vi "get voltage range ring.vi"(8 "error in (no error)":errorcluster caption="에러 입력(에러 없음)", 11 "DW7914 입력":refnum<class "DW7914.lvclass">) -> (0 "error out":errorcluster caption="에러 출력", 1 "caption":string="VD Clamp", 2 "strings & values":T1=[{"String"="0.00V", "Value"=0.0}, {"String"="0.04V", "Value"=0.04}, {"String"="0.08V", "Value"=0.08}, {"String"="0.12V", "Value"=0.12}, {"String"="0.16V", "Value"=0.16}, {"String"="0.20V", "Value"=0.2}, {"String"="0.24V", "Value"=0.24}, {"String"="0.28V", "Value"=0.28}, {"String"="0.32V", "Value"=0.32}, {"String"="0.36V", "Value"=0.36}, {"String"="0.40V", "Value"=0.4}, {"String"="0.44V", "Value"=0.44}, {"String"="0.48V", "Value"=0.48}, {"String"="0.52V", "Value"=0.52}, {"String"="0.56V", "Value"=0.56}, {"String"="0.60V", "Value"=0.6}, {"String"="0.64V", "Value"=0.64}, {"String"="0.68V", "Value"=0.68}, {"String"="0.72V", "Value"=0.72}, {"String"="0.76V", "Value"=0.76}, {"String"="0.80V", "Value"=0.8}, {"String"="0.84V", "Value"=0.84}, {"String"="0.88V", "Value"=0.88}, {"String"="0.92V", "Value"=0.92}, {"String"="0.96V", "Value"=0.96}, {"String"="1.00V", "Value"=1.0}, {"String"="1.04V", "Value"=1.04}, {"String"="1.08V", "Value"=1.08}, {"String"="1.12V", "Value"=1.12}, {"String"="1.16V", "Value"=1.16}, {"String"="1.20V", "Value"=1.2}, {"String"="1.24V", "Value"=1.24}, {"String"="1.28V", "Value"=1.28}, {"String"="1.32V", "Value"=1.32}, {"String"="1.36V", "Value"=1.36}, {"String"="1.40V", "Value"=1.4}, {"String"="1.44V", "Value"=1.44}, {"String"="1.48V", "Value"=1.48}, {"String"="1.52V", "Value"=1.52}, {"String"="1.56V", "Value"=1.56}, {"String"="1.60V", "Value"=1.6}, {"String"="1.64V", "Value"=1.64}, {"String"="1.68V", "Value"=1.68}, {"String"="1.72V", "Value"=1.72}, {"String"="1.76V", "Value"=1.76}, {"String"="1.80V", "Value"=1.8}, {"String"="1.84V", "Value"=1.84}, {"String"="1.88V", "Value"=1.88}, {"String"="1.92V", "Value"=1.92}, {"String"="1.96V", "Value"=1.96}, {"String"="2.00V", "Value"=2.0}, {"String"="2.04V", "Value"=2.04}, {"String"="2.08V", "Value"=2.08}, {"String"="2.12V", "Value"=2.12}, {"String"="2.16V", "Value"=2.16}, {"String"="2.20V", "Value"=2.2}, {"String"="2.24V", "Value"=2.24}, {"String"="2.28V", "Value"=2.28}, {"String"="2.32V", "Value"=2.32}, {"String"="2.36V", "Value"=2.36}, {"String"="2.40V", "Value"=2.4}, {"String"="2.44V", "Value"=2.44}, {"String"="2.48V", "Value"=2.48}, {"String"="2.52V", "Value"=2.52}, {"String"="2.56V", "Value"=2.56}, {"String"="2.60V", "Value"=2.6}, {"String"="2.64V", "Value"=2.64}, {"String"="2.68V", "Value"=2.68}, {"String"="2.72V", "Value"=2.72}, {"String"="2.76V", "Value"=2.76}, {"String"="2.80V", "Value"=2.8}, {"String"="2.84V", "Value"=2.84}, {"String"="2.88V", "Value"=2.88}, {"String"="2.92V", "Value"=2.92}, {"String"="2.96V", "Value"=2.96}, {"String"="3.00V", "Value"=3.0}, {"String"="3.04V", "Value"=3.04}, {"String"="3.08V", "Value"=3.08}, {"String"="3.12V", "Value"=3.12}, {"String"="3.16V", "Value"=3.16}, {"String"="3.20V", "Value"=3.2}, {"String"="3.24V", "Value"=3.24}, {"String"="3.28V", "Value"=3.28}, {"String"="3.32V", "Value"=3.32}, {"String"="3.36V", "Value"=3.36}, {"String"="3.40V", "Value"=3.4}, {"String"="3.44V", "Value"=3.44}, {"String"="3.48V", "Value"=3.48}, {"String"="3.52V", "Value"=3.52}, {"String"="3.56V", "Value"=3.56}, {"String"="3.60V", "Value"=3.6}, {"String"="3.64V", "Value"=3.64}, {"String"="3.68V", "Value"=3.68}, {"String"="3.72V", "Value"=3.72}, {"String"="3.76V", "Value"=3.76}, {"String"="3.80V", "Value"=3.8}, {"String"="3.84V", "Value"=3.84}, {"String"="3.88V", "Value"=3.88}, {"String"="3.92V", "Value"=3.92}, {"String"="3.96V", "Value"=3.96}, {"String"="4.00V", "Value"=4.0}, {"String"="4.04V", "Value"=4.04}, {"String"="4.08V", "Value"=4.08}, {"String"="4.12V", "Value"=4.12}, {"String"="4.16V", "Value"=4.16}, {"String"="4.20V", "Value"=4.2}, {"String"="4.24V", "Value"=4.24}, {"String"="4.28V", "Value"=4.28}, {"String"="4.32V", "Value"=4.32}, {"String"="4.36V", "Value"=4.36}, {"String"="4.40V", "Value"=4.4}, {"String"="4.44V", "Value"=4.44}, {"String"="4.48V", "Value"=4.48}, {"String"="4.52V", "Value"=4.52}, {"String"="4.56V", "Value"=4.56}, {"String"="4.60V", "Value"=4.6}, {"String"="4.64V", "Value"=4.64}, {"String"="4.68V", "Value"=4.68}, {"String"="4.72V", "Value"=4.72}, {"String"="4.76V", "Value"=4.76}, {"String"="4.80V", "Value"=4.8}, {"String"="4.84V", "Value"=4.84}, {"String"="4.88V", "Value"=4.88}, {"String"="4.92V", "Value"=4.92}, {"String"="4.96V", "Value"=4.96}, {"String"="5.00V", "Value"=5.0}, {"String"="5.04V", "Value"=5.04}, {"String"="5.08V", "Value"=5.08}, {"String"="5.12V", "Value"=5.12}, {"String"="5.16V", "Value"=5.16}, {"String"="5.20V", "Value"=5.2}, {"String"="5.24V", "Value"=5.24}, {"String"="5.28V", "Value"=5.28}, {"String"="5.32V", "Value"=5.32}, {"String"="5.36V", "Value"=5.36}, {"String"="5.40V", "Value"=5.4}, {"String"="5.44V", "Value"=5.44}, {"String"="5.48V", "Value"=5.48}, {"String"="5.52V", "Value"=5.52}, {"String"="5.56V", "Value"=5.56}, {"String"="5.60V", "Value"=5.6}, {"String"="5.64V", "Value"=5.64}, {"String"="5.68V", "Value"=5.68}, {"String"="5.72V", "Value"=5.72}, {"String"="5.76V", "Value"=5.76}, {"String"="5.80V", "Value"=5.8}, {"String"="5.84V", "Value"=5.84}, {"String"="5.88V", "Value"=5.88}, {"String"="5.92V", "Value"=5.92}, {"String"="5.96V", "Value"=5.96}, {"String"="6.00V", "Value"=6.0}, {"String"="6.04V", "Value"=6.04}, {"String"="6.08V", "Value"=6.08}, {"String"="6.12V", "Value"=6.12}, {"String"="6.16V", "Value"=6.16}, {"String"="6.20V", "Value"=6.2}, {"String"="6.24V", "Value"=6.24}, {"String"="6.28V", "Value"=6.28}, {"String"="6.32V", "Value"=6.32}, {"String"="6.36V", "Value"=6.36}, {"String"="6.40V", "Value"=6.4}, {"String"="6.44V", "Value"=6.44}, {"String"="6.48V", "Value"=6.48}, {"String"="6.52V", "Value"=6.52}, {"String"="6.56V", "Value"=6.56}, {"String"="6.60V", "Value"=6.6}, {"String"="6.64V", "Value"=6.64}, {"String"="6.68V", "Value"=6.68}, {"String"="6.72V", "Value"=6.72}, {"String"="6.76V", "Value"=6.76}, {"String"="6.80V", "Value"=6.8}, {"String"="6.84V", "Value"=6.84}, {"String"="6.88V", "Value"=6.88}, {"String"="6.92V", "Value"=6.92}, {"String"="6.96V", "Value"=6.96}, {"String"="7.00V", "Value"=7.0}, {"String"="7.04V", "Value"=7.04}, {"String"="7.08V", "Value"=7.08}, {"String"="7.12V", "Value"=7.12}, {"String"="7.16V", "Value"=7.16}, {"String"="7.20V", "Value"=7.2}, {"String"="7.24V", "Value"=7.24}, {"String"="7.28V", "Value"=7.28}, {"String"="7.32V", "Value"=7.32}, {"String"="7.36V", "Value"=7.36}, {"String"="7.40V", "Value"=7.4}, {"String"="7.44V", "Value"=7.44}, {"String"="7.48V", "Value"=7.48}, {"String"="7.52V", "Value"=7.52}, {"String"="7.56V", "Value"=7.56}, {"String"="7.60V", "Value"=7.6}, {"String"="7.64V", "Value"=7.64}, {"String"="7.68V", "Value"=7.68}, {"String"="7.72V", "Value"=7.72}, {"String"="7.76V", "Value"=7.76}, {"String"="7.80V", "Value"=7.8}, {"String"="7.84V", "Value"=7.84}, {"String"="7.88V", "Value"=7.88}, {"String"="7.92V", "Value"=7.92}, {"String"="7.96V", "Value"=7.96}, {"String"="8.00V", "Value"=8.0}, {"String"="8.04V", "Value"=8.04}, {"String"="8.08V", "Value"=8.08}, {"String"="8.12V", "Value"=8.12}, {"String"="8.16V", "Value"=8.16}, {"String"="8.20V", "Value"=8.2}, {"String"="8.24V", "Value"=8.24}, {"String"="8.28V", "Value"=8.28}, {"String"="8.32V", "Value"=8.32}, {"String"="8.36V", "Value"=8.36}, {"String"="8.40V", "Value"=8.4}, {"String"="8.44V", "Value"=8.44}, {"String"="8.48V", "Value"=8.48}, {"String"="8.52V", "Value"=8.52}, {"String"="8.56V", "Value"=8.56}, {"String"="8.60V", "Value"=8.6}, {"String"="8.64V", "Value"=8.64}, {"String"="8.68V", "Value"=8.68}, {"String"="8.72V", "Value"=8.72}, {"String"="8.76V", "Value"=8.76}, {"String"="8.80V", "Value"=8.8}, {"String"="8.84V", "Value"=8.84}, {"String"="8.88V", "Value"=8.88}, {"String"="8.92V", "Value"=8.92}, {"String"="8.96V", "Value"=8.96}, {"String"="9.00V", "Value"=9.0}, {"String"="9.04V", "Value"=9.04}, {"String"="9.08V", "Value"=9.08}, {"String"="9.12V", "Value"=9.12}, {"String"="9.16V", "Value"=9.16}, {"String"="9.20V", "Value"=9.2}, {"String"="9.24V", "Value"=9.24}, {"String"="9.28V", "Value"=9.28}, {"String"="9.32V", "Value"=9.32}, {"String"="9.36V", "Value"=9.36}, {"String"="9.40V", "Value"=9.4}, {"String"="9.44V", "Value"=9.44}, {"String"="9.48V", "Value"=9.48}, {"String"="9.52V", "Value"=9.52}, {"String"="9.56V", "Value"=9.56}, {"String"="9.60V", "Value"=9.6}, {"String"="9.64V", "Value"=9.64}, {"String"="9.68V", "Value"=9.68}, {"String"="9.72V", "Value"=9.72}, {"String"="9.76V", "Value"=9.76}, {"String"="9.80V", "Value"=9.8}, {"String"="9.84V", "Value"=9.84}, {"String"="9.88V", "Value"=9.88}, {"String"="9.92V", "Value"=9.92}, {"String"="9.96V", "Value"=9.96}, {"String"="10.00V", "Value"=10.0}, {"String"="10.04V", "Value"=10.04}, {"String"="10.08V", "Value"=10.08}, {"String"="10.12V", "Value"=10.12}, {"String"="10.16V", "Value"=10.16}, {"String"="10.20V", "Value"=10.2}], 3 "DW7914 출력":refnum<class "DW7914.lvclass">, 4 "read value":dbl)   [LabVIEW 2020, in "DW7914.lvclass"]
uses:
  DW7914.lvclass
  <vilib>/Utility/miscctls.llb/LVStringsAndValuesArrayTypeDef_DBL.ctl
  Haptic IC/Haptic IC.lvclass/Haptic IC.ctl
  SubVIs/I2C/Instance VIs/(SubVI)I2C_8Bit-8Bit_Read_Single.vi
  Haptic IC/Haptic IC.lvclass
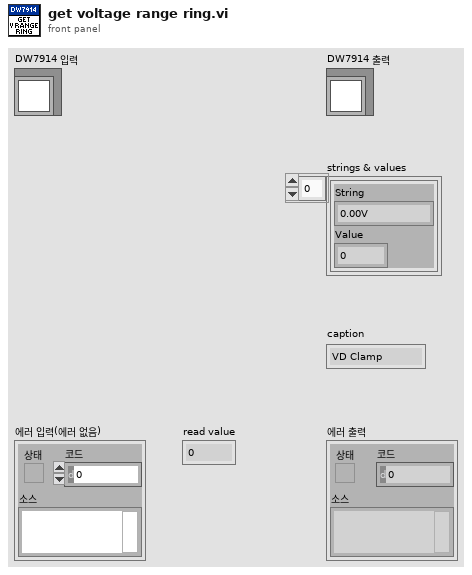
[diagram p1: front panel]
types:
  T1 = typedef "LVStringsAndValuesArrayTypeDef_DBL.ctl" = cluster{"String":string, "Value":dbl}[]
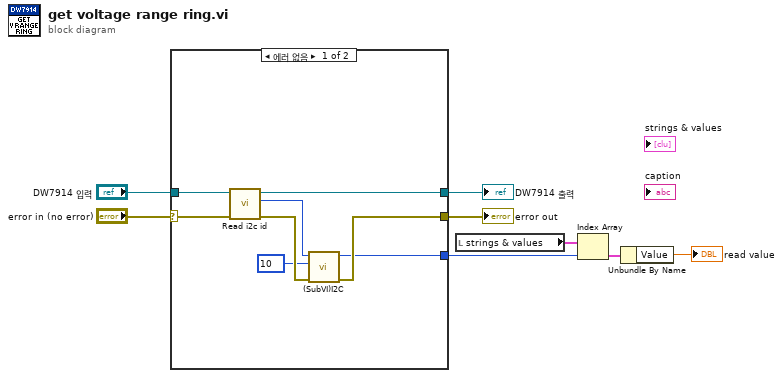
[diagram p0: block diagram]
diagram:
  n1 = case shown="에러 없음" "error in (no error)" {
    selector: "error in (no error)" -> [w15 w17]
    tunnel: "DW7914 입력" -> [w16 w18]
    tunnel: [w14 w18] -> w7
    tunnel: [w10 w17] -> w8
    tunnel: [w9 _] -> w3
    frame No Error {
      n2 = call "Read i2c id.vi"("error in (no error)"=w15, "Haptic IC 입력"=w16) -> ("error out"=w13:errorcluster, "i2c id"=w12:u8, "Haptic IC 출력"=w14:refnum<class "DW7914.lvclass">)  [unwired: 7 in]
      n3 = call-poly "(SubVI)I2C.vi"("error in (no error)"=w13, "Address"=u8 10, "ID"=w12) -> ("error out"=w10:errorcluster, "Read Data"=w9:u8)  [unwired: 6 in, 1 out]
    }
    frame Error {
    }
  }
  "error out" <- w8
  "DW7914 출력" <- w7
  n4 = local read "strings & values"() -> (w1:T1)
  n5 = Index Array(array=w1, index=w3) -> (element=w2:cluster{"String":string, "Value":dbl})
  n6 = Unbundle By Name(w2) -> ("Value"=→"read value":dbl)
